vi "BarLIV_SearchAndPlot_Main_v1.vi"() -> ()   [LabVIEW 2017]
uses:
  <vilib>/Utility/NIReport.llb/NI_report.lvclass
panel:
  in  "Date Selection":i32[](listbox)
  out "Input selection subarray":string[][](array[string])
  out "Selected Wafer ID":string[](array[string])
  out "Selected Bar WO":string[](array[string])
  out "Selected Bar SN":string[](array[string])
  out "Selected Test Date":string[](array[string])
  out "Input selection Items":string[][](array[string])
  in  "Tab Control":enum32{"Raw Data", "Selected Data"}(tab)
  out "Raw Bar Table Data":string[][](array[string])=[["1", "3/22/2019", "30101152", "DM17-20                  ", "                         ", "31 emitters/Pass", "30", "0.06", "1.375", "933.884", "37.774", "0.145"], ["2", "3/22/2019", "30101152", "DM17-20                  ", "                         ", "31 emitters/Pass", "60", "24.48", "1.414", "935.13", "41.871", "28.854"], ["3", "3/22/2019", "30101152", "DM17-20                  ", "                         ", "31 emitters/Pass", "90", "57.61", "1.445", "935.9", "44.404", "44.298"], ["4", "3/22/2019", "30101152", "DM17-20                  ", "                         ", "31 emitters/Pass", "120", "91.3", "1.475", "936.78", "47.298", "51.582"], ["5", "3/22/2019", "30101152", "DM17-20                  ", "                         ", "31 emitters/Pass", "150", "125", "1.504", "937.76", "50.522", "55.408"], ["6", "3/22/2019", "30101152", "DM17-20                  ", "                         ", "31 emitters/Pass", "180", "158.3", "1.532", "938.84", "54.075", "57.405"], ["7", "3/22/2019", "30101152", "DM17-20                  ", "                         ", "31 emitters/Pass", "210", "191.3", "1.56", "939.97", "57.792", "58.394"], ["8", "3/22/2019", "30101152", "DM17-20                  ", "                         ", "31 emitters/Pass", "240", "222.8", "1.587", "941.25", "62.002", "58.496"], ["9", "3/22/2019", "30101152", "DM17-20                  ", "                         ", "31 emitters/Pass", "270", "253.6", "1.613", "942.63", "66.542", "58.231"], ["10", "3/22/2019", "30101152", "DM17-20                  ", "                         ", "31 emitters/Pass", "300", "282.9", "1.639", "944.11", "71.41", "57.535"], ["11", "3/22/2019", "30101152", "DM17-20                  ", "                         ", "31 emitters/Pass", "330", "311.2", "1.664", "945.73", "76.739", "56.672"], ["12", "3/22/2019", "30101562", "DM17-20                  ", "                         ", "Pass", "30", "0.18", "1.374", "934.413", "37.888", "0.437"], ["13", "3/22/2019", "30101562", "DM17-20                  ", "                         ", "Pass", "60", "25.92", "1.413", "935.59", "41.76", "30.573"], ["14", "3/22/2019", "30101562", "DM17-20                  ", "                         ", "Pass", "90", "59.94", "1.443", "936.37", "44.326", "46.154"], ["15", "3/22/2019", "30101562", "DM17-20                  ", "                         ", "Pass", "120", "94.3", "1.473", "937.19", "47.023", "53.349"], ["16", "3/22/2019", "30101562", "DM17-20                  ", "                         ", "Pass", "150", "128.7", "1.502", "938.12", "50.083", "57.124"], ["17", "3/22/2019", "30101562", "DM17-20                  ", "                         ", "Pass", "180", "162.8", "1.53", "939.14", "53.438", "59.114"], ["18", "3/22/2019", "30101562", "DM17-20                  ", "                         ", "Pass", "210", "196.5", "1.557", "940.27", "57.155", "60.097"], ["19", "3/22/2019", "30101562", "DM17-20                  ", "                         ", "Pass", "240", "229.2", "1.584", "941.5", "61.201", "60.29"], ["20", "3/22/2019", "30101562", "DM17-20                  ", "                         ", "Pass", "270", "261", "1.61", "942.83", "65.576", "60.041"], ["21", "3/22/2019", "30101562", "DM17-20                  ", "                         ", "Pass", "300", "291.7", "1.635", "944.21", "70.115", "59.47"], ["22", "3/22/2019", "30101562", "DM17-20                  ", "                         ", "Pass", "330", "320.8", "1.659", "945.83", "75.444", "58.597"], ["23", "3/22/2019", "30101566", "DM17-20                  ", "                         ", "Fail", "30", "0.14", "1.375", "934.203", "37.774", "0.339"], ["24", "3/22/2019", "30101566", "DM17-20                  ", "                         ", "Fail", "60", "25.11", "1.413", "935.39", "41.68", "29.618"], ["25", "3/22/2019", "30101566", "DM17-20                  ", "                         ", "Fail", "90", "58.98", "1.444", "936.11", "44.048", "45.383"], ["26", "3/22/2019", "30101566", "DM17-20                  ", "                         ", "Fail", "120", "93.3", "1.473", "936.93", "46.745", "52.783"], ["27", "3/22/2019", "30101566", "DM17-20                  ", "                         ", "Fail", "150", "127.7", "1.502", "937.91", "49.969", "56.68"], ["28", "3/22/2019", "30101566", "DM17-20                  ", "                         ", "Fail", "180", "161.8", "1.53", "938.84", "53.028", "58.751"], ["29", "3/22/2019", "30101566", "DM17-20                  ", "                         ", "Fail", "210", "195.3", "1.558", "939.97", "56.745", "59.692"], ["30", "3/22/2019", "30101566", "DM17-20                  ", "                         ", "Fail", "240", "228.2", "1.584", "941.04", "60.265", "60.027"], ["31", "3/22/2019", "30101566", "DM17-20                  ", "                         ", "Fail", "270", "260.1", "1.61", "942.37", "64.64", "59.834"], ["32", "3/22/2019", "30101566", "DM17-20                  ", "                         ", "Fail", "300", "290.9", "1.635", "943.75", "69.18", "59.307"], ["33", "3/22/2019", "30101566", "DM17-20                  ", "                         ", "Fail", "330", "320.2", "1.66", "945.28", "74.212", "58.452"], ["34", "3/22/2019", "30101586", "DM17-20                  ", "                         ", "Pass", "30", "0.12", "1.375", "934.057", "37.55", "0.291"], ["35", "3/22/2019", "30101586", "DM17-20                  ", "                         ", "Pass", "60", "24.93", "1.415", "935.23", "41.41", "29.364"], ["36", "3/22/2019", "30101586", "DM17-20                  ", "                         ", "Pass", "90", "58.6", "1.447", "935.95", "43.778", "44.997"], ["37", "3/22/2019", "30101586", "DM17-20                  ", "                         ", "Pass", "120", "92.9", "1.478", "936.78", "46.509", "52.379"], ["38", "3/22/2019", "30101586", "DM17-20                  ", "                         ", "Pass", "150", "127.3", "1.507", "937.71", "49.568", "56.315"], ["39", "3/22/2019", "30101586", "DM17-20                  ", "                         ", "Pass", "180", "161.3", "1.537", "938.68", "52.759", "58.303"], ["40", "3/22/2019", "30101586", "DM17-20                  ", "                         ", "Pass", "210", "194.7", "1.565", "939.76", "56.311", "59.242"], ["41", "3/22/2019", "30101586", "DM17-20                  ", "                         ", "Pass", "240", "227.6", "1.593", "940.89", "60.028", "59.531"], ["42", "3/22/2019", "30101586", "DM17-20                  ", "                         ", "Pass", "270", "259.4", "1.62", "942.12", "64.075", "59.305"], ["43", "3/22/2019", "30101586", "DM17-20                  ", "                         ", "Pass", "300", "290.1", "1.647", "943.49", "68.581", "58.713"], ["44", "3/22/2019", "30101586", "DM17-20                  ", "                         ", "Pass", "330", "319.4", "1.673", "945.02", "73.614", "57.853"], ["45", "3/22/2019", "30101731", "DM17-20                  ", "                         ", "31 emitters/Pass", "30", "0.18", "1.375", "933.644", "37.885", "0.436"], ["46", "3/22/2019", "30101731", "DM17-20                  ", "                         ", "31 emitters/Pass", "60", "24.92", "1.415", "934.87", "41.92", "29.352"], ["47", "3/22/2019", "30101731", "DM17-20                  ", "                         ", "31 emitters/Pass", "90", "58.52", "1.446", "935.64", "44.453", "44.967"], ["48", "3/22/2019", "30101731", "DM17-20                  ", "                         ", "31 emitters/Pass", "120", "92.7", "1.475", "936.47", "47.183", "52.373"], ["49", "3/22/2019", "30101731", "DM17-20                  ", "                         ", "31 emitters/Pass", "150", "126.8", "1.505", "937.45", "50.407", "56.168"], ["50", "3/22/2019", "30101731", "DM17-20                  ", "                         ", "31 emitters/Pass", "180", "160.3", "1.533", "938.48", "53.795", "58.092"], ["51", "3/22/2019", "30101731", "DM17-20                  ", "                         ", "31 emitters/Pass", "210", "192.9", "1.561", "939.55", "57.314", "58.845"], ["52", "3/22/2019", "30101731", "DM17-20                  ", "                         ", "31 emitters/Pass", "240", "224.9", "1.588", "940.73", "61.196", "59.01"], ["53", "3/22/2019", "30101731", "DM17-20                  ", "                         ", "31 emitters/Pass", "270", "255.6", "1.614", "942.06", "65.571", "58.653"], ["54", "3/22/2019", "30101731", "DM17-20                  ", "                         ", "31 emitters/Pass", "300", "285.6", "1.64", "943.54", "70.439", "58.049"], ["55", "3/22/2019", "30101731", "DM17-20                  ", "                         ", "31 emitters/Pass", "330", "313.9", "1.665", "945.12", "75.637", "57.13"]]
  out "Data Selected (<10)":string[][](array[string])
  in  "Bar SN Selection":i32[](listbox)
  in  "Bar WO Selection":i32[](listbox)
  in  "Wafer ID Selection":i32[](listbox)=[2]
  out "BarWO Select Output Subarry":string[][](array[string])=[["03/22/2019", "201", "1", "1"], ["03/22/2019", "201", "1", "2"], ["03/22/2019", "204", "3", "2"]]
  out "WaferID Select Output Subarry":string[][](array[string])=[["03/22/2019", "201", "1", "1"], ["03/22/2019", "201", "1", "2"], ["03/22/2019", "204", "2", "1"], ["03/22/2019", "204", "3", "2"], ["03/22/2018", "205", "4", ""], ["03/22/2018", "206", "5", ""], ["03/22/2018", "207", "7", ""], ["03/22/2018", "208", "7", ""]]
  in  "Stop and Plot":bool
  in  "Input File Name":string="report_1"
  in  "File Directory to Save Report":path=path "D:/LabVIEW_prog/Trumpf_Database_Connect/Report_output"
  in  "Excel Template":path=path "D:/LabVIEW_prog/Trumpf_Database_Connect/Bar_LIV_ExcelTemp.xlsx"
  out "Select Data":string[][](array[string])=[["23", "3/22/2019", "30101566", "DM17-20                  ", "                         ", "Fail", "30", "0.14", "1.375", "934.203", "37.774", "0.339"], ["24", "3/22/2019", "30101566", "DM17-20                  ", "                         ", "Fail", "60", "25.11", "1.413", "935.39", "41.68", "29.618"], ["25", "3/22/2019", "30101566", "DM17-20                  ", "                         ", "Fail", "90", "58.98", "1.444", "936.11", "44.048", "45.383"], ["26", "3/22/2019", "30101566", "DM17-20                  ", "                         ", "Fail", "120", "93.3", "1.473", "936.93", "46.745", "52.783"], ["27", "3/22/2019", "30101566", "DM17-20                  ", "                         ", "Fail", "150", "127.7", "1.502", "937.91", "49.969", "56.68"], ["28", "3/22/2019", "30101566", "DM17-20                  ", "                         ", "Fail", "180", "161.8", "1.53", "938.84", "53.028", "58.751"], ["29", "3/22/2019", "30101566", "DM17-20                  ", "                         ", "Fail", "210", "195.3", "1.558", "939.97", "56.745", "59.692"], ["30", "3/22/2019", "30101566", "DM17-20                  ", "                         ", "Fail", "240", "228.2", "1.584", "941.04", "60.265", "60.027"], ["31", "3/22/2019", "30101566", "DM17-20                  ", "                         ", "Fail", "270", "260.1", "1.61", "942.37", "64.64", "59.834"], ["32", "3/22/2019", "30101566", "DM17-20                  ", "                         ", "Fail", "300", "290.9", "1.635", "943.75", "69.18", "59.307"], ["33", "3/22/2019", "30101566", "DM17-20                  ", "                         ", "Fail", "330", "320.2", "1.66", "945.28", "74.212", "58.452"]]
  in  "Finish Selection":bool
  out "Error Out":errorcluster
  in  "Error In":errorcluster
  # "Bar LIV Selection From RD Database - Chao Gong"
  # "Note: \n1) Select test date, bar SN, work order, and wafer ID. (Leave it blank for all selection). \n2) Click finish selection.\n3) Click stop to save excel file and generate plotting report\n4) No more 10 selection a time (Excel template runs out)"
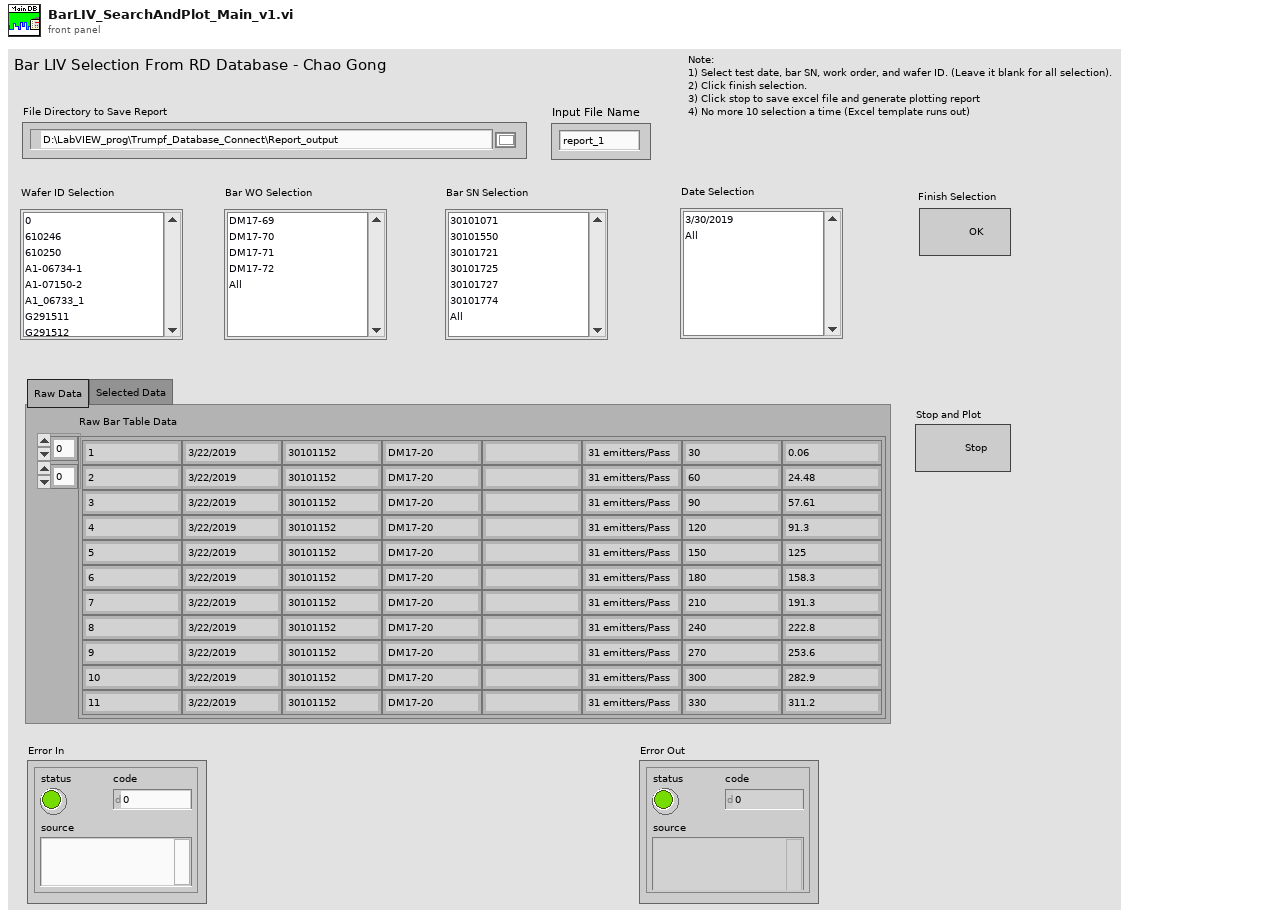
[diagram p1: front panel]
types:
  T1 = enum16{"Standard Report", "HTML", "Word", "Excel"}
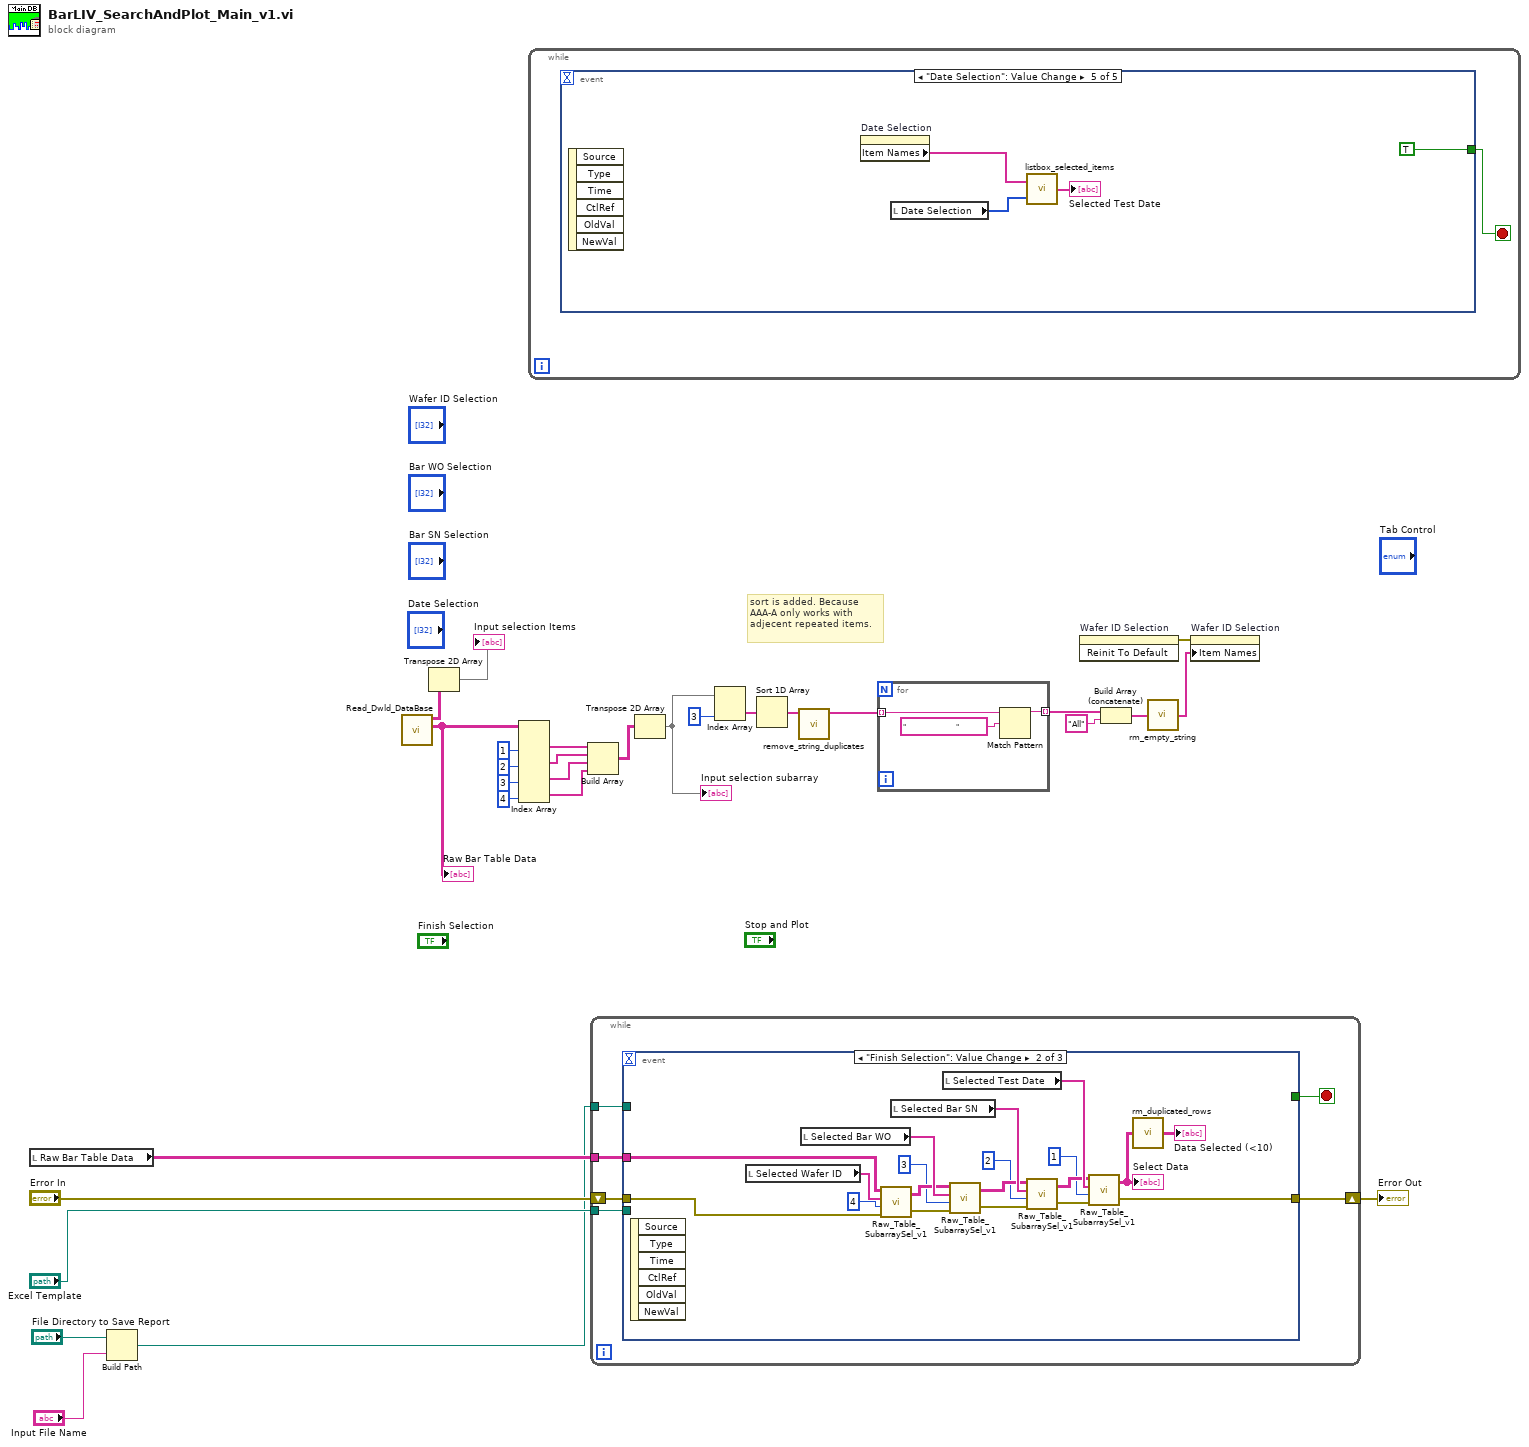
[diagram p0: block diagram]
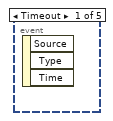
[diagram p2: hidden frame]
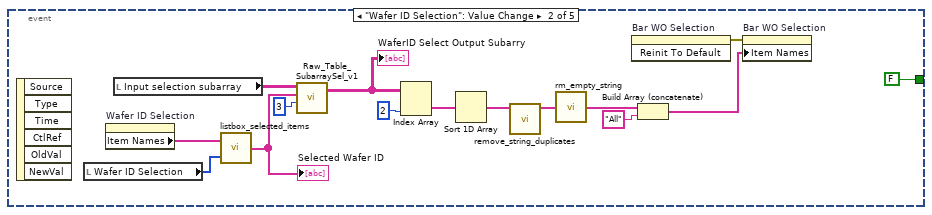
[diagram p3: hidden frame]
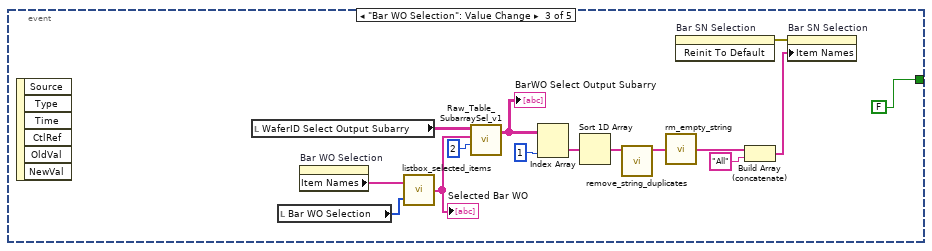
[diagram p4: hidden frame]
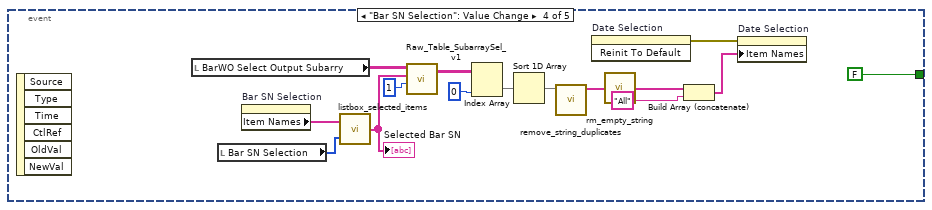
[diagram p5: hidden frame]
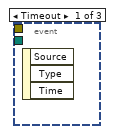
[diagram p6: hidden frame]
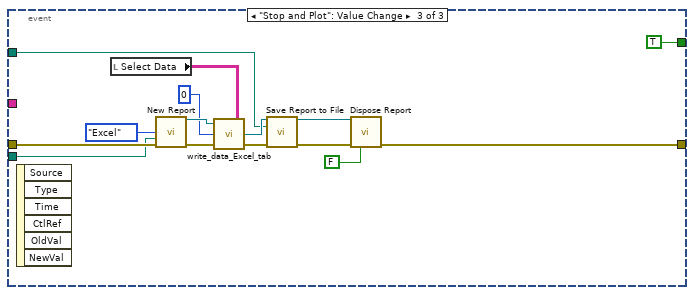
[diagram p7: hidden frame]
diagram:
  # "sort is added. Because AAA-A only works with adjecent repeated items."
  n1 = local read "Raw Bar Table Data"() -> (w29:string[][])
  n2 = Build Path(base path="File Directory to Save Report", name or relative path="Input File Name") -> (appended path=w24:path)
  n3 = call "Read_Dwld_DataBase.vi"() -> ("Output Data"=w11:string[][], "Output selection string"=w13:string[][])  [unwired: 4 in, 2 out]
  "Raw Bar Table Data" <- w11
  n4 = Transpose 2D Array(2D array=w13) -> (transposed array=→"Input selection Items":string[][])
  n5 = Index Array(array=w11, index (col) #1=1 ("disabled index (col)"), index (col) #2=2 ("index (col)"), index (col) #3=3 ("index (col)"), index (col) #4=4 ("index (col)")) -> (element #1=w6:string[], element #2=w5:string[], element #3=w4:string[], element #4=w3:string[])  [unwired: 4 in]
  n6 = while {
    stop <- w30 stop-if-true
    n7 = event shown="[4] \"Date Selection\": Value Change" {
      selector: _ -> [_ _ _ _ _]
      dyn-events: _ -> [_ _ _ _ _]
      timeout: _ -> [_ _ _ _ _]
      tunnel: [_ FALSE ("stop") FALSE ("stop") FALSE ("stop") TRUE ("stop")] -> w30
      event Timeout {
        n8 = event-data() -> ()  [unwired: 1 in, 3 out]
      }
      event "Wafer ID Selection": Value Change {
        n9 = event-data() -> ()  [unwired: 1 in, 6 out]
        n10 = local read "Wafer ID Selection"() -> (w34:i32[])
        n11 = property on="Wafer ID Selection" class="LstBox (strict)"() -> ("Item Names"=w35:string[])  [unwired: 2 in, 2 out]
        n12 = local read "Input selection subarray"() -> (w45:string[][])
        n13 = call "listbox_selected_items.vi"("Selected item number"=w34, "All items"=w35) -> ("Selected items"=w33:string[])
        "Selected Wafer ID" <- w33
        n14 = call "Raw_Table_SubarraySel_v1.vi"("Column Index"=3, "String to compare"=w33, "Raw Bar Table Data"=w45) -> ("Selected Output"=w42:string[][])  [unwired: 1 in, 1 out]
        "WaferID Select Output Subarry" <- w42
        n15 = Index Array(array=w42, index (col)=2 ("disabled index (col)")) -> (element=w32:string[])  [unwired: 1 in]
        n16 = Sort 1D Array(array=w32) -> (sorted array=w31:string[])
        n17 = call "remove_string_duplicates.vi"("In"=w31) -> ("Out"=w38:string[])  [unwired: 10 in]
        n18 = call "rm_empty_string.vi"("Array"=w38) -> ("String output"=w40:string[])
        n19 = invoke on="Bar WO Selection" class="LstBox (strict)" method="Reinit To Default"() -> (error out=w36:errorcluster)  [unwired: 3 in, 2 out]
        n20 = Build Array (concatenate)(w40, "All") -> (w37:string[])
        n21 = property on="Bar WO Selection" class="LstBox (strict)"(error in=w36, "Item Names"=w37) -> ()  [unwired: 1 in, 2 out]
      }
      event "Bar WO Selection": Value Change {
        n22 = event-data() -> ()  [unwired: 1 in, 6 out]
        n23 = local read "WaferID Select Output Subarry"() -> (w60:string[][])
        n24 = local read "Bar WO Selection"() -> (w49:i32[])
        n25 = property on="Bar WO Selection" class="LstBox (strict)"() -> ("Item Names"=w50:string[])  [unwired: 2 in, 2 out]
        n26 = call "listbox_selected_items.vi"("Selected item number"=w49, "All items"=w50) -> ("Selected items"=w48:string[])
        "Selected Bar WO" <- w48
        n27 = call "Raw_Table_SubarraySel_v1.vi"("Column Index"=2, "String to compare"=w48, "Raw Bar Table Data"=w60) -> ("Selected Output"=w58:string[][])  [unwired: 1 in, 1 out]
        "BarWO Select Output Subarry" <- w58
        n28 = Index Array(array=w58, index (col)=1 ("disabled index (col)")) -> (element=w47:string[])  [unwired: 1 in]
        n29 = Sort 1D Array(array=w47) -> (sorted array=w46:string[])
        n30 = call "remove_string_duplicates.vi"("In"=w46) -> ("Out"=w53:string[])  [unwired: 10 in]
        n31 = call "rm_empty_string.vi"("Array"=w53) -> ("String output"=w55:string[])
        n32 = invoke on="Bar SN Selection" class="LstBox (strict)" method="Reinit To Default"() -> (error out=w51:errorcluster)  [unwired: 3 in, 2 out]
        n33 = Build Array (concatenate)(w55, "All") -> (w52:string[])
        n34 = property on="Bar SN Selection" class="LstBox (strict)"(error in=w51, "Item Names"=w52) -> ()  [unwired: 1 in, 2 out]
      }
      event "Bar SN Selection": Value Change {
        n35 = event-data() -> ()  [unwired: 1 in, 6 out]
        n36 = local read "BarWO Select Output Subarry"() -> (w75:string[][])
        n37 = local read "Bar SN Selection"() -> (w66:i32[])
        n38 = property on="Bar SN Selection" class="LstBox (strict)"() -> ("Item Names"=w67:string[])  [unwired: 2 in, 2 out]
        n39 = call "listbox_selected_items.vi"("Selected item number"=w66, "All items"=w67) -> ("Selected items"=w65:string[])
        "Selected Bar SN" <- w65
        n40 = call "Raw_Table_SubarraySel_v1.vi"("Column Index"=1, "String to compare"=w65, "Raw Bar Table Data"=w75) -> ("Selected Output"=w73:string[][])  [unwired: 1 in, 1 out]
        n41 = Index Array(array=w73, index (col)=0 ("disabled index (col)")) -> (element=w64:string[])  [unwired: 1 in]
        n42 = Sort 1D Array(array=w64) -> (sorted array=w63:string[])
        n43 = call "remove_string_duplicates.vi"("In"=w63) -> ("Out"=w71:string[])  [unwired: 10 in]
        n44 = invoke on="Date Selection" class="LstBox (strict)" method="Reinit To Default"() -> (error out=w61:errorcluster)  [unwired: 3 in, 2 out]
        n45 = call "rm_empty_string.vi"("Array"=w71) -> ("String output"=w70:string[])
        n46 = Build Array (concatenate)(w70, "All") -> (w62:string[])
        n47 = property on="Date Selection" class="LstBox (strict)"(error in=w61, "Item Names"=w62) -> ()  [unwired: 1 in, 2 out]
      }
      event "Date Selection": Value Change {
        n48 = event-data() -> ()  [unwired: 1 in, 6 out]
        n49 = property on="Date Selection" class="LstBox (strict)"() -> ("Item Names"=w76:string[])  [unwired: 2 in, 2 out]
        n50 = local read "Date Selection"() -> (w78:i32[])
        n51 = call "listbox_selected_items.vi"("Selected item number"=w78, "All items"=w76) -> ("Selected items"=→"Selected Test Date":string[])
      }
    }
  }
  n52 = Build Array(w6, w5, w4, w3) -> (w2:string[][])
  n53 = while {
    tunnel: w29 -> [w85]
    shift-right: [w83] -> w27
    shift-left: "Error In" -> [w84]
    tunnel: "Excel Template" -> [w82]
    tunnel: w24 -> [w81]
    stop <- w80 stop-if-true
    n54 = event shown="[1] \"Finish Selection\": Value Change" {
      selector: _ -> [_ _ _]
      dyn-events: _ -> [_ _ _]
      timeout: _ -> [_ _ _]
      tunnel: w85 -> [_ w88 _]
      tunnel: w84 -> [_ w93 w117]
      tunnel: [_ w89 w112] -> w83
      tunnel: w82 -> [_ _ w115]
      tunnel: w81 -> [_ _ w109]
      tunnel: [_ _ TRUE ("Stop Search and Plot")] -> w80
      event Timeout {
        n55 = event-data() -> ()  [unwired: 1 in, 3 out]
      }
      event "Finish Selection": Value Change {
        n56 = event-data() -> ()  [unwired: 1 in, 6 out]
        n57 = local read "Selected Wafer ID"() -> (w104:string[])
        n58 = local read "Selected Bar WO"() -> (w102:string[])
        n59 = call "Raw_Table_SubarraySel_v1.vi"("error in (no error)"=w93, "Column Index"=4, "String to compare"=w104, "Raw Bar Table Data"=w88) -> ("error out"=w92:errorcluster, "Selected Output"=w101:string[][])
        n60 = local read "Selected Bar SN"() -> (w99:string[])
        n61 = local read "Selected Test Date"() -> (w96:string[])
        n62 = call "Raw_Table_SubarraySel_v1.vi"("error in (no error)"=w92, "Column Index"=3, "String to compare"=w102, "Raw Bar Table Data"=w101) -> ("error out"=w91:errorcluster, "Selected Output"=w98:string[][])
        n63 = call "Raw_Table_SubarraySel_v1.vi"("error in (no error)"=w91, "Column Index"=2, "String to compare"=w99, "Raw Bar Table Data"=w98) -> ("error out"=w90:errorcluster, "Selected Output"=w95:string[][])
        n64 = call "Raw_Table_SubarraySel_v1.vi"("error in (no error)"=w90, "Column Index"=1, "String to compare"=w96, "Raw Bar Table Data"=w95) -> ("error out"=w89:errorcluster, "Selected Output"=w87:string[][])
        "Select Data" <- w87
        n65 = call "rm_duplicated_rows.vi"("Select Data"=w87) -> ("Output Data"=→"Data Selected (<10)":string[][])
      }
      event "Stop and Plot": Value Change {
        n66 = event-data() -> ()  [unwired: 1 in, 6 out]
        n67 = local read "Select Data"() -> (w119:string[][])
        n68 = call <vilib>:"New Report.vi"("report type"=T1."Excel", "template (empty)"=w115, "error in (no error)"=w117) -> ("report out"=w118:refnum<class "NI_report.lvclass">, "error out"=w116:errorcluster)  [unwired: 3 in, 8 out]
        n69 = call "write_data_Excel_tab.vi"("text data"=w119, "error in (no error)"=w116, "worksheet index (0)"=0, "report in"=w118) -> ("error out"=w108:errorcluster, "report out"=w110:refnum<class "NI_report.lvclass">)
        n70 = call-dynamic "Save Report to File.vi"("report in"=w110, "report file path"=w109, "error in (no error)"=w108) -> ("report out"=w107:refnum<class "NI_report.lvclass">, "error out"=w106:errorcluster)  [unwired: 11 in]
        n71 = call-dynamic "Dispose Report.vi"("report in"=w107, "error in (no error)"=w106, "close report? (T)"=FALSE) -> ("error out"=w112:errorcluster)  [unwired: 12 in]
      }
    }
  }
  "Error Out" <- w27
  n72 = Transpose 2D Array(2D array=w2) -> (transposed array=w1:string[][])
  "Input selection subarray" <- w1
  n73 = Index Array(array=w1, index (col)=3 ("disabled index (col)")) -> (element=w16:string[])  [unwired: 1 in]
  n74 = Sort 1D Array(array=w16) -> (sorted array=w15:string[])
  n75 = call "remove_string_duplicates.vi"("In"=w15) -> ("Out"=w20:string[])  [unwired: 10 in]
  n76 = for {
    tunnel: w20 -> [w122] mode=indexing
    tunnel: [w120] -> w19 mode=indexing
    n77 = Match Pattern(string=w122, regular expression="                         ") -> (before substring=w120:string)  [unwired: 1 in, 3 out]
  }
  n78 = invoke on="Wafer ID Selection" class="LstBox (strict)" method="Reinit To Default"() -> (error out=w17:errorcluster)  [unwired: 3 in, 2 out]
  n79 = Build Array (concatenate)(w19, "All") -> (w18:string[])
  n80 = call "rm_empty_string.vi"("Array"=w18) -> ("String output"=w14:string[])
  n81 = property on="Wafer ID Selection" class="LstBox (strict)"(error in=w17, "Item Names"=w14) -> ()  [unwired: 1 in, 2 out]
